vi "DriveOver.vi"(2 "Parameter String":string="near", 3 "Reinit":bool) -> (0 "Error Out":errorcluster, 1 "Increment":bool)   [LabVIEW 2020]
doc: "The swerve drive base will translate in the field-centric X direction until it reaches the CHARGING STATION. Then it will move up the ramp and balance using the pitch feedback from the IMU.\n\nParameters:\n1. \"near\" or \"far\" to indicate which side the robot is coming from in relation to the driver station"
uses:
  fecc16b4-9204-47e7-b057-41e41d998ae7.vi
  0fe48bd2-3b49-4c8c-82c6-f24528f2b59d.vi
  9c209fce-094d-437e-8f6c-1b0f354aa5a3.vi
  3ab4cadb-8a01-4273-86b8-f239e16545bb.vi
  a7ed37be-f2ea-4a93-9181-94187c83a0c7.vi
  d3142cce-3259-45a8-b5d9-00d720d151ea.vi
  SafeParser_String.vi
  GlobalDriverStationData.vi
  GlobalDriverStationCommands.vi
  GlobalPoseAndTargeting.vi
panel:
  in  "Down ramp power":dbl=0.1 format="%#_13g"
  in  "Up ramp power":dbl=0.3
  in  "Movement stopped threshold":dbl=2.0
  in  "Power Integration per Loop":dbl=0.001 format="%#_13g"
  in  "Power to Drive to Ramp":dbl=0.3 format="%#_13g"
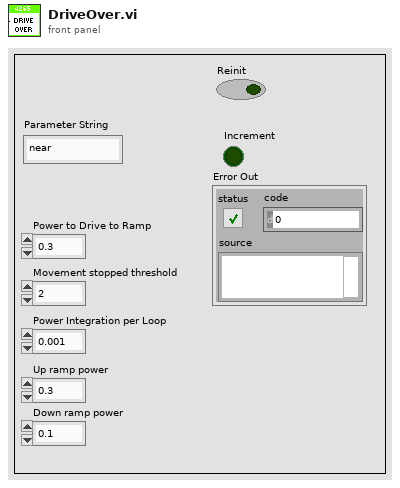
[diagram p1: front panel]
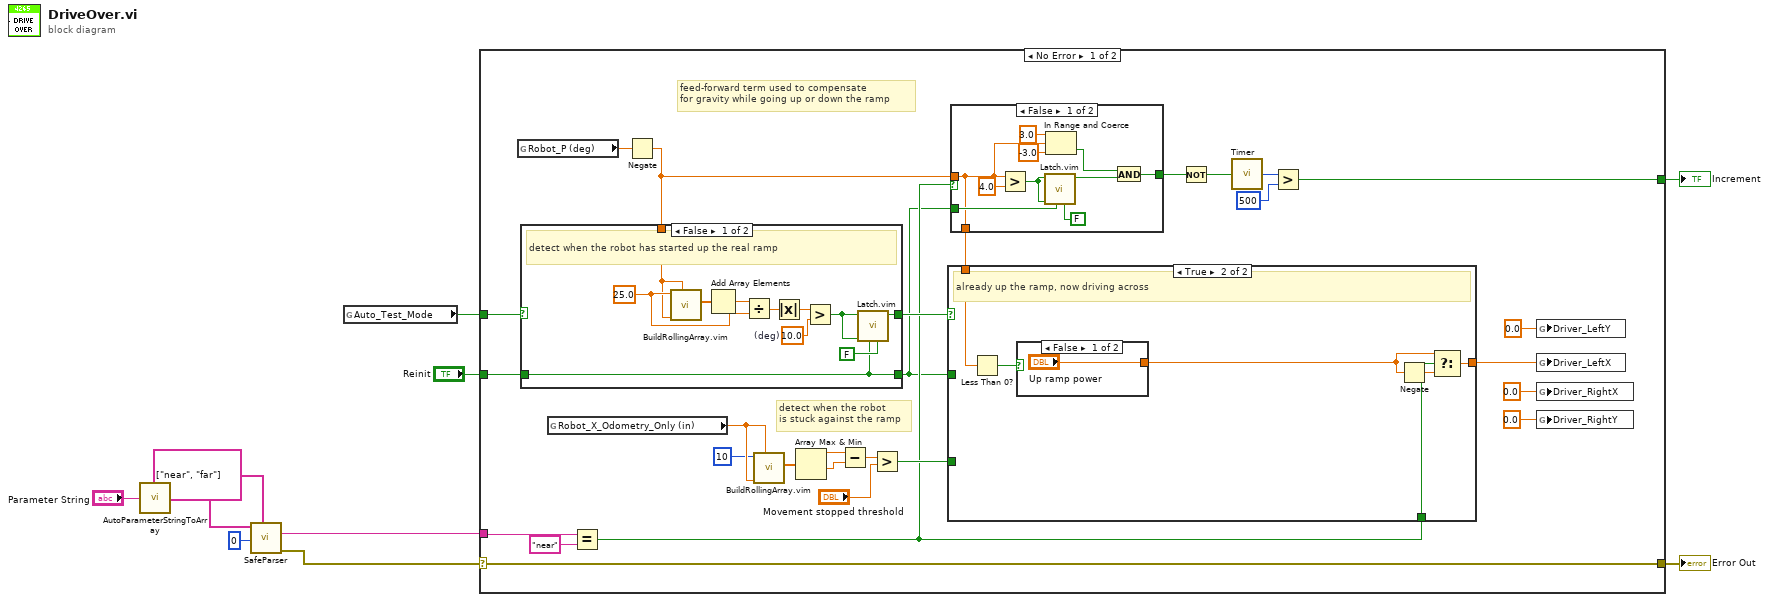
[diagram p0: block diagram]
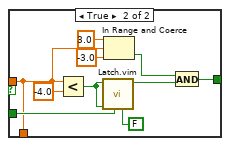
[diagram p2: hidden frame]
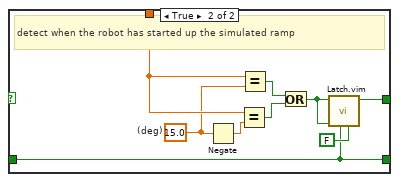
[diagram p3: hidden frame]
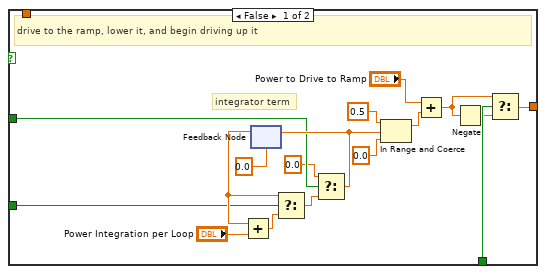
[diagram p4: hidden frame]
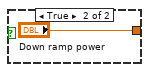
[diagram p5: hidden frame]
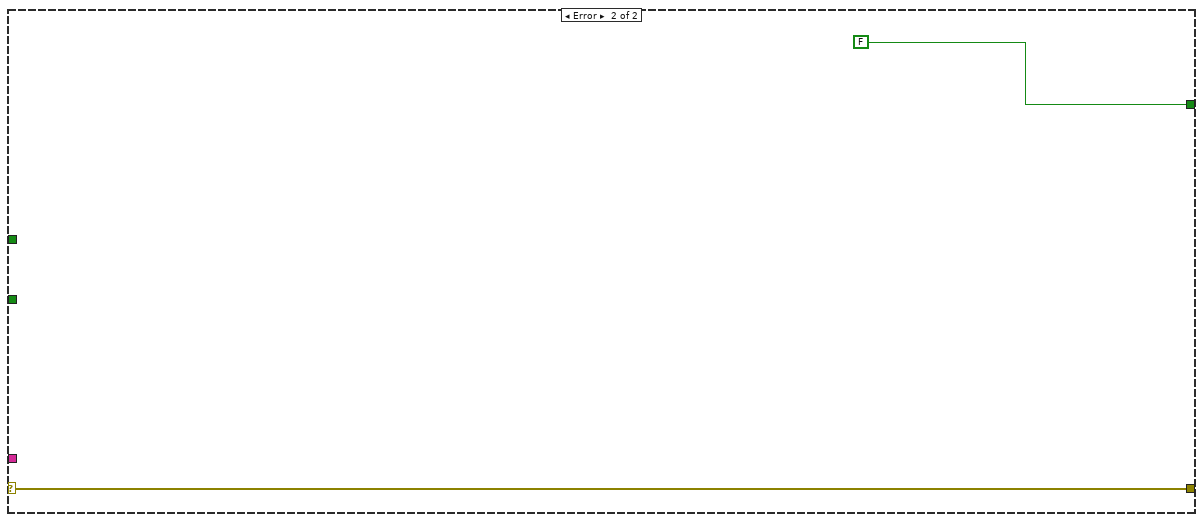
[diagram p6: hidden frame]
diagram:
  n1 = call "AutoParameterStringToArray.vi"("Parameter String"="Parameter String") -> ("Parsed Parameters"=w7:string[])
  n2 = call-poly "SafeParser.vi"("Allowed Values"=string[] ["near", "far"], "Array Index"=0 ("Parameter Index"), "String Array"=w7) -> ("Error Out"=w2:errorcluster, "Typecast Value"=w6:string)  [unwired: 7 in]
  n3 = global read "GlobalDriverStationData.vi" "Auto_Test_Mode"() -> (w1:bool)
  n4 = case shown="No Error" w2 {
    selector: w2 -> [w38 w105]
    tunnel: [w11 FALSE] -> w4
    tunnel: "Reinit" -> [w30 _]
    tunnel: [w38 w105] -> w9
    tunnel: w6 -> [w35 _]
    tunnel: w1 -> [w29 _]
    frame No Error {
      # "detect when the robot\nis stuck against the ramp"
      # "feed-forward term used to compensate\nfor gravity while going up or down the ramp"
      n5 = global read "GlobalPoseAndTargeting.vi" "Robot_P (deg)"() -> (w36:dbl)
      n6 = global read "GlobalPoseAndTargeting.vi" "Robot_X_Odometry_Only (in)"() -> (w28:dbl)
      n7 = Equal?(x=w35, y="near") -> (x = y?=w19:bool)
      n8 = Negate(x=w36) -> (-x=w18:dbl)
      n9 = case shown="False" w29 {
        tunnel: [w62 w76] -> w31
        tunnel: w18 -> [w61 w75]
        tunnel: w30 -> [w59 w77]
        tunnel: [w59 w77] -> w16
        frame False {
          w65 = 10.0  # (deg)
          w67 = 25.0 ("Number of Elements")
          # "detect when the robot has started up the real ramp"
          n10 = call "BuildRollingArray.vim"("New Value"=w61, "Initial Value"=w61, "Number of Elements"=w67) -> ("Current Array"=w69:dbl[])  [unwired: 8 in]
          n11 = Add Array Elements(numeric array=w69) -> (sum=w68:dbl)
          n12 = Divide(x=w68, y=w67) -> (x/y=w66:dbl)
          n13 = Absolute Value(x=w66) -> (abs(x)=w60:dbl)
          n14 = Greater?(x=w60, y=w65) -> (0:w63:bool)
          n15 = call "Latch.vim"("Default Value"=FALSE, "Reset"=w59, "Latch Signal"=w63, "Latch Value"=w63) -> ("Latched"=w62:bool)  [unwired: 7 in]
        }
        frame True {
          w70 = 15.0  # (deg)
          # "detect when the robot has started up the simulated ramp"
          n16 = Negate(x=w70) -> (-x=w71:dbl)
          n17 = Equal?(x=w75, y=w71) -> (x = y?=w73:bool)
          n18 = Equal?(x=w75, y=w70) -> (x = y?=w74:bool)
          n19 = Or(x=w74, y=w73) -> (x .or. y?=w72:bool)
          n20 = call "Latch.vim"("Default Value"=FALSE, "Reset"=w77, "Latch Signal"=w72, "Latch Value"=w72) -> ("Latched"=w76:bool)  [unwired: 7 in]
        }
      }
      n21 = call "BuildRollingArray.vim"("New Value"=w28, "Initial Value"=w28, "Number of Elements"=10) -> ("Current Array"=w27:dbl[])  [unwired: 8 in]
      n22 = Array Max & Min(array=w27) -> (max value=w26:dbl, min value=w25:dbl)  [unwired: 2 out]
      n23 = Subtract(x=w26, y=w25) -> (x-y=w24:dbl)
      n24 = Greater?(x=w24, y="Movement stopped threshold") -> (0:w22:bool)
      n25 = case shown="False" w19 {
        tunnel: w18 -> [w39 w52]
        tunnel: [w39 w52] -> w17
        tunnel: w16 -> [w40 w54]
        tunnel: [w42 w49] -> w15
        frame False {
          n26 = Greater?(x=w39, y=4.0) -> (0:w48:bool)
          n27 = call "Latch.vim"("Default Value"=FALSE, "Reset"=w40, "Latch Signal"=w48, "Latch Value"=w48) -> ("Latched"=w46:bool)  [unwired: 7 in]
          n28 = In Range and Coerce(upper limit=3.0, x=w39, lower limit=-3.0) -> (In Range?=w45:bool)  [unwired: 1 out]
          n29 = And(x=w45, y=w46) -> (x .and. y?=w42:bool)
        }
        frame True {
          n30 = Less?(x=w52, y=-4.0) -> (x < y?=w57:bool)
          n31 = call "Latch.vim"("Default Value"=FALSE, "Reset"=w54, "Latch Signal"=w57, "Latch Value"=w57) -> ("Latched"=w55:bool)  [unwired: 7 in]
          n32 = In Range and Coerce(upper limit=3.0, x=w52, lower limit=-3.0) -> (In Range?=w53:bool)  [unwired: 1 out]
          n33 = And(x=w53, y=w55) -> (x .and. y?=w49:bool)
        }
      }
      n34 = case shown="True" w31 {
        tunnel: [w80 w99] -> w20
        tunnel: w17 -> [_ w100]
        tunnel: w19 -> [w91 w98]
        tunnel: w16 -> [w85 _]
        tunnel: w22 -> [w79 _]
        frame False {
          # "integrator term"
          # "drive to the ramp, lower it, and begin driving up it"
          n35 = feedback #1(0.0) -> (w93:dbl)
          n36 = Add(x=w93, y="Power Integration per Loop") -> (x+y=w94:dbl)
          n37 = Select(t=w93, s=w79, f=w94) -> (s? t:f=w88:dbl)
          n38 = Select(t=0.0, s=w85, f=w88) -> (s? t:f=w86:dbl)
          n39 = feedback-in #1(w86) -> ()
          n40 = In Range and Coerce(upper limit=0.5, x=w86, lower limit=0.0) -> (coerced(x)=w87:dbl)  [unwired: 1 out]
          n41 = Add(x="Power to Drive to Ramp", y=w87) -> (x+y=w82:dbl)
          n42 = Negate(x=w82) -> (-x=w81:dbl)
          n43 = Select(t=w82, s=w91, f=w81) -> (s? t:f=w80:dbl)
        }
        frame True {
          # "already up the ramp, now driving across"
          n44 = Less Than 0?(x=w100) -> (x < 0?=w101:bool)
          n45 = case shown="False" w101 {
            tunnel: ["Up ramp power" "Down ramp power"] -> w97
            frame False {
            }
            frame True {
            }
          }
          n46 = Negate(x=w97) -> (-x=w96:dbl)
          n47 = Select(t=w97, s=w98, f=w96) -> (s? t:f=w99:dbl)
        }
      }
      n48 = Not(x=w15) -> (.not. x?=w13:bool)
      n49 = call "Timer.vi"("Reset Timer"=w13) -> ("Time (ms)"=w14:u32)
      n50 = Greater?(x=w14, y=u32 500) -> (0:w11:bool)
      n51 = global write "GlobalDriverStationCommands.vi" "Driver_LeftY"(0.0 ("Driver_LeftY")) -> ()
      n52 = global write "GlobalDriverStationCommands.vi" "Driver_LeftX"(w20) -> ()
      n53 = global write "GlobalDriverStationCommands.vi" "Driver_RightX"(0.0 ("Driver_RightX")) -> ()
      n54 = global write "GlobalDriverStationCommands.vi" "Driver_RightY"(0.0 ("Driver_RightX")) -> ()
    }
    frame Error {
    }
  }
  "Increment" <- w4
  "Error Out" <- w9
